vi "ADI_IMU_ADIS16448_Reset.vi"(8 "error in":errorcluster, 11 "ADI IMU DevRef":T1={"DevStatus"={"status"=FALSE, "code"=0, "source"=""}, "Handle"=27, "SPI Bus"=enum."SPI MXP", "Device Found"=TRUE, "Device Ready"=FALSE, "Yaw Axis"=enum."Z", "AHRS Algorithm"=enum."Complementary", "Serial"=118, "Lot ID 2"=5379, "Lot ID 1"=118, "Bytes Per Sample"=0, "Calibrate On Open?"=FALSE}) -> (0 "error out":errorcluster, 3 "ADI IMU DevRef Out":T1={"DevStatus"={"status"=FALSE, "code"=0, "source"=""}, "Handle"=27, "SPI Bus"=enum."SPI MXP", "Device Found"=TRUE, "Device Ready"=FALSE, "Yaw Axis"=enum."Z", "AHRS Algorithm"=enum."Complementary", "Serial"=118, "Lot ID 2"=5379, "Lot ID 1"=118, "Bytes Per Sample"=0, "Calibrate On Open?"=FALSE})   [LabVIEW 2017, in "ADIS16448_IMU.lvlib"]
doc: "Resets the accumulated angles to zero in software. This VI does NOT electrically reset the ADI MXP IMU or reset the calibration."
uses:
  ADIS16448_IMU.lvlib
  ADI_IMU_ADIS16448_IMUDevRef.ctl
  <vilib>/Rock Robotics/SystemInterfaces/spilib/spi_bus.ctl
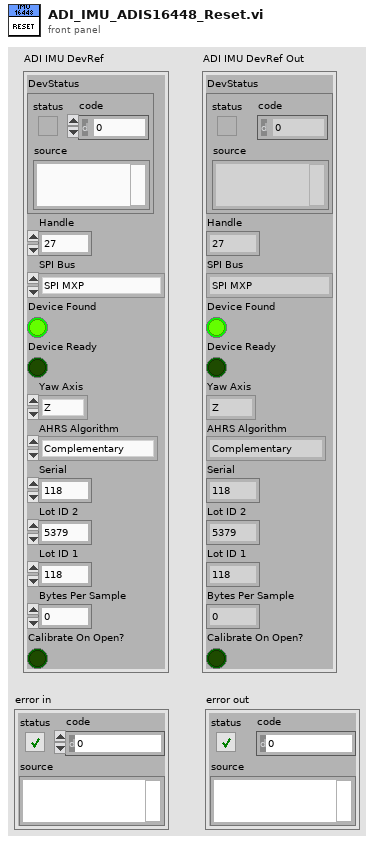
[diagram p1: front panel]
types:
  T1 = typedef "ADIS16448_IMU.lvlib/ADI_IMU_ADIS16448_IMUDevRef.ctl" = cluster{"DevStatus":errorcluster, "Handle":i32, "SPI Bus":T2, "Device Found":bool, "Device Ready":bool, "Yaw Axis":enum16{"X", "Y", "Z"}, "AHRS Algorithm":enum16{"Complementary", "Madgwick"}, "Serial":u16, "Lot ID 2":u16, "Lot ID 1":u16, "Bytes Per Sample":u16, "Calibrate On Open?":bool}
  T2 = typedef "spi_bus.ctl" = enum16{"SPI On-Board, CS0", "SPI On-Board, CS1", "SPI On-Board, CS2", "SPI On-Board, CS3", "SPI MXP", "Invalid"}
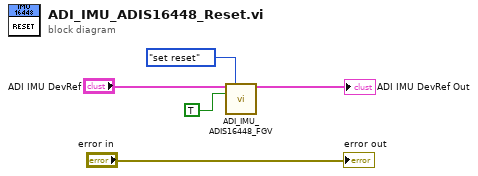
[diagram p0: block diagram]
diagram:
  n1 = call "ADI_IMU_ADIS16448_FGV.vi"("ADI IMU DevRef"="ADI IMU DevRef", "Operation"=enum16{"set", "get", "set reset"}."set reset", "Reset"=TRUE) -> ("ADI IMU DevRef Out"=→"ADI IMU DevRef Out":T1)  [unwired: 6 in, 6 out]
  "error out" <- "error in"
